vi "DriveParams_KCubeInertial.vi"(6 "MaxVoltage":i32, 9 "StepAcceleration":i32, 10 "StepRate":i32, 11 ".NET Refnum in":refnum<k24>) -> (3 "Cluster":T1)   [LabVIEW 2019]
doc: "drive parameters for absolute position movements for inertial motor"
uses:
  D:/Victor Sun/optical trap control/Kinesis/Thorlabs.MotionControl.KCube.InertialMotorCLI.dll
  Kinesis/Thorlabs.MotionControl.KCube.InertialMotorCLI.dll
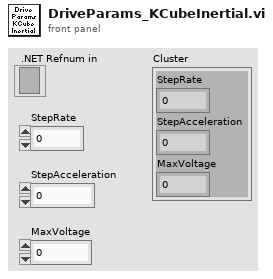
[diagram p1: front panel]
types:
  T1 = cluster{"StepRate":i32, "StepAcceleration":i32, "MaxVoltage":i32}
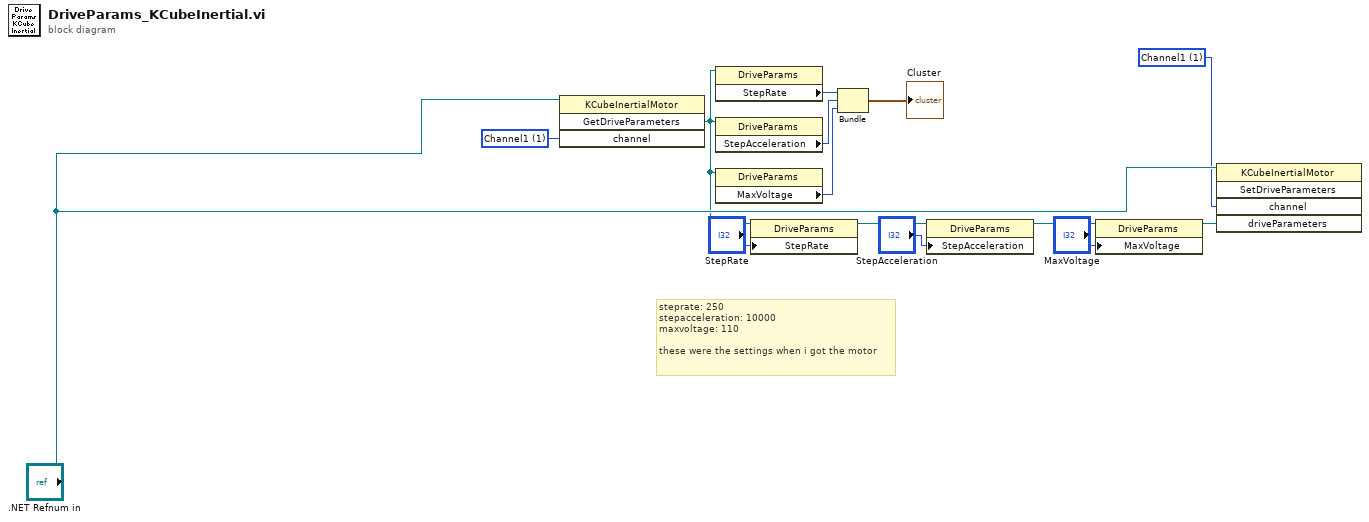
[diagram p0: block diagram]
diagram:
  w6 = 1 items=["Channel1"=1, "Channel2"=2, "Channel3"=3, "Channel4"=4] ("channel")
  w1 = 1 items=["Channel1"=1, "Channel2"=2, "Channel3"=3, "Channel4"=4] ("channel")
  # "steprate: 250\nstepacceleration: 10000\nmaxvoltage: 110\n\nthese were the settings when i got the motor"
  n1 = invoke class="KCubeInertialMotor" method="GetDriveParameters"(reference=".NET Refnum in", "channel"=w1) -> ("GetDriveParameters"=w2:refnum<k24>)  [unwired: 2 in, 3 out]
  n2 = property class="DriveParams"(reference=w2) -> ("StepRate"=w13:i32)  [unwired: 1 in, 2 out]
  n3 = property class="DriveParams"(reference=w2) -> ("StepAcceleration"=w11:i32)  [unwired: 1 in, 2 out]
  n4 = property class="DriveParams"(reference=w2) -> ("MaxVoltage"=w12:i32)  [unwired: 1 in, 2 out]
  n5 = property class="DriveParams"(reference=w2, "StepRate"="StepRate") -> (reference out=w3:refnum<k24>)  [unwired: 1 in, 1 out]
  n6 = Bundle("StepRate"=w13, "StepAcceleration"=w11, "MaxVoltage"=w12) -> (→"Cluster":T1)  [unwired: 1 in]
  n7 = property class="DriveParams"(reference=w3, "StepAcceleration"="StepAcceleration") -> (reference out=w4:refnum<k24>)  [unwired: 1 in, 1 out]
  n8 = property class="DriveParams"(reference=w4, "MaxVoltage"="MaxVoltage") -> (reference out=w5:refnum<k24>)  [unwired: 1 in, 1 out]
  n9 = invoke class="KCubeInertialMotor" method="SetDriveParameters"(reference=".NET Refnum in", "channel"=w6, "driveParameters"=w5) -> ()  [unwired: 2 in, 5 out]
